vi "Connect Channels (Single).vi"(8 "error in (no error)":errorcluster, 9 "channel 2":string, 10 "channel 1":string, 11 "SLSC Switch in":refnum<class "SLSC Switch.lvclass">) -> (0 "error out":errorcluster, 3 "SLSC Switch out":refnum<class "SLSC Switch.lvclass">)   [LabVIEW 2015, in "SLSC Switch.lvlib" / "SLSC Switch.lvclass"]
doc: "Creates a path between channel 1 and channel 2. SLSC-SWITCH calculates and uses the shortest path between the two channels."
uses:
  SLSC Switch.lvclass
  slscsl/slscsl.lvclass
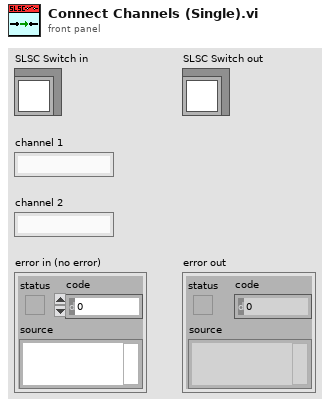
[diagram p1: front panel]
types:
  T1 = typedef "SLSC Switch.lvlib/slscsl.lvclass/SwitchActionsArray.ctl" = T2[]
  T2 = typedef "SLSC Switch.lvlib/slscsl.lvclass/SwitchAction.ctl" = cluster{"index":i32, "RelayAction":T3}
  T3 = typedef "SLSC Switch.lvlib/slscsl.lvclass/RelayAction.ctl" = u32
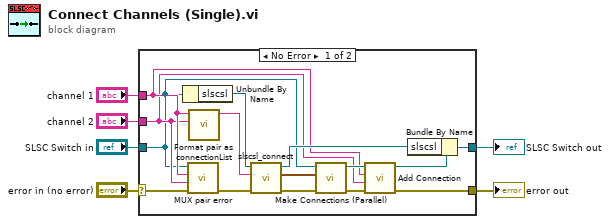
[diagram p0: block diagram]
diagram:
  n1 = case shown="No Error" "error in (no error)" {
    selector: "error in (no error)" -> [w11 w23]
    tunnel: [w16 w23] -> w5
    tunnel: "SLSC Switch in" -> [w7 w22]
    tunnel: "channel 1" -> [w9 _]
    tunnel: "channel 2" -> [w8 _]
    tunnel: [w14 w22] -> w1
    frame No Error {
      n2 = Unbundle By Name(w7) -> ("slscsl"=w20:refnum<class "slscsl.lvclass">)
      n3 = call "MUX pair error.vi"("error in (no error)"=w11, "channel 2"=w8, "channel 1"=w9, "SLSC Switch in"=w7) -> ("error out"=w10:errorcluster)  [unwired: 7 in]
      n4 = call "Format pair as connectionList.vi"("channel in"=w8, "channel 1"=w9) -> ("connectionList"=w19:string)  [unwired: 9 in]
      n5 = call "slscsl_connect.vi"("error in (no error)"=w10, "connectionList"=w19, "slscsl in"=w20) -> ("error out"=w21:errorcluster, "switchActionsArray"=w12:T1, "slscsl out"=w13:refnum<class "slscsl.lvclass">)  [unwired: 6 in]
      n6 = call "Make Connections (Parallel).vi"("error in (no error)"=w21, "switchActionsArray"=w12, "SLSC Switch in"=w7) -> ("error out"=w18:errorcluster, "SLSC Switch out"=w17:refnum<class "SLSC Switch.lvclass">)  [unwired: 7 in]
      n7 = call "Add Connection.vi"("error in (no error)"=w18, "channel 2"=w8, "channel 1"=w9, "SLSC Switch in"=w17) -> ("error out"=w16:errorcluster, "SLSC Switch out"=w15:refnum<class "SLSC Switch.lvclass">)  [unwired: 6 in]
      n8 = Bundle By Name(cluster=w15, "slscsl"=w13) -> (w14:refnum<class "SLSC Switch.lvclass">)
    }
    frame Error {
    }
  }
  "error out" <- w5
  "SLSC Switch out" <- w1
